vi "NI-Digital Burst I2C.vi"() -> ()   [LabVIEW 2024]
doc: "Overview\nDemonstrates how to use the NI-Digital Pattern Driver API to create and configure an instrument session and to burst a pattern on the digital pattern instrument using a start trigger."
uses:
  <instrlib>/niDigital/niDigital.llb/niDigital Write Static Pin State.ctl
  <instrlib>/niDigital/niDigital.llb/niDigital Selected Function.ctl
  <instrlib>/niDigital/niDigital.llb/niDigital Load Specifications Levels and Timing (Single).vi
  <instrlib>/niDigital/niDigital.llb/niDigital Write Source Waveform (Site Unique U32).vi
  <instrlib>/niDigital/niDigital.llb/niDigital Burst Pattern (Burst Only).vi
  <instrlib>/Semi Device Control/Utils/DIO Pin State.ctl
  <instrlib>/Semi Device Control/Semiconductor Device Control.lvclass
panel:
  in  "Tab Control":enum32{"SDC on", "Digital Low Level"}(tab)
  in  "Write SDC":bool
  in  "stop":bool
  in  "Register UID":string="CTRL_REG1"
  out "Register Value":u64
  in  "Write Value SDC":u64 format="%.0b"
  in  "Read SDC":bool
  in  "stop SDC":bool
  in  "Register Adress":u64 format="%.0x"
  out "Register Value Low Level":u32
  in  "Digital Pattern Resource":refnum<k15>="HSD_6571_C01_S02" caption="resource name"
  in  "Write Data":u64 format="%.0x"
  in  "Write Button LL":bool
  in  "Read Button LL":bool
  out "error out":errorcluster
  # "Overview\nDemonstrates how to use the NI-Digital Pattern Driver API to create and configure an instrument session and to burst a pattern on the digital pattern instrument using a start trigger.\n\nInstructions\n1. Use the resource name control to select the digital pattern instrument. Ensure that the instrument name in the PinMap.pinmap file matches the resource name of the digital pattern instrument. The default value for the resource name is \"PXI1Slot2,PXI1Slot3\".\n2. Use the start trigger mode tab control to select the start trigger mode to use. The active tab determines the configured start trigger at run time. Some tabs include additional configuration options.\n3. Run the VI.\n4. To run on hardware deselect Simulate?  and modify the resource name as appropriate."
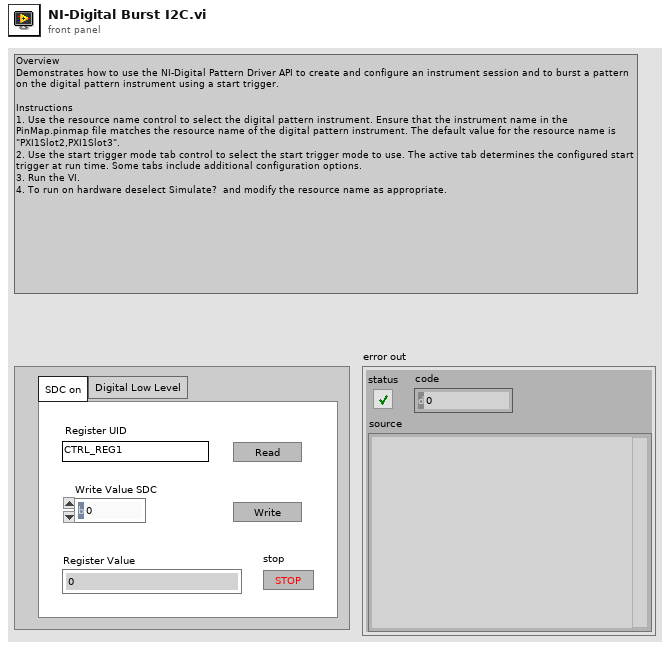
[diagram p1: front panel]
types:
  T1 = typedef "Semiconductor Device Control.lvclass/DIO Pin State.ctl" = enum16{"Low", "High", "Term"}
  T2 = typedef "niDigital Write Static Pin State.ctl" = u8
  T3 = typedef "niDigital Selected Function.ctl" = i32
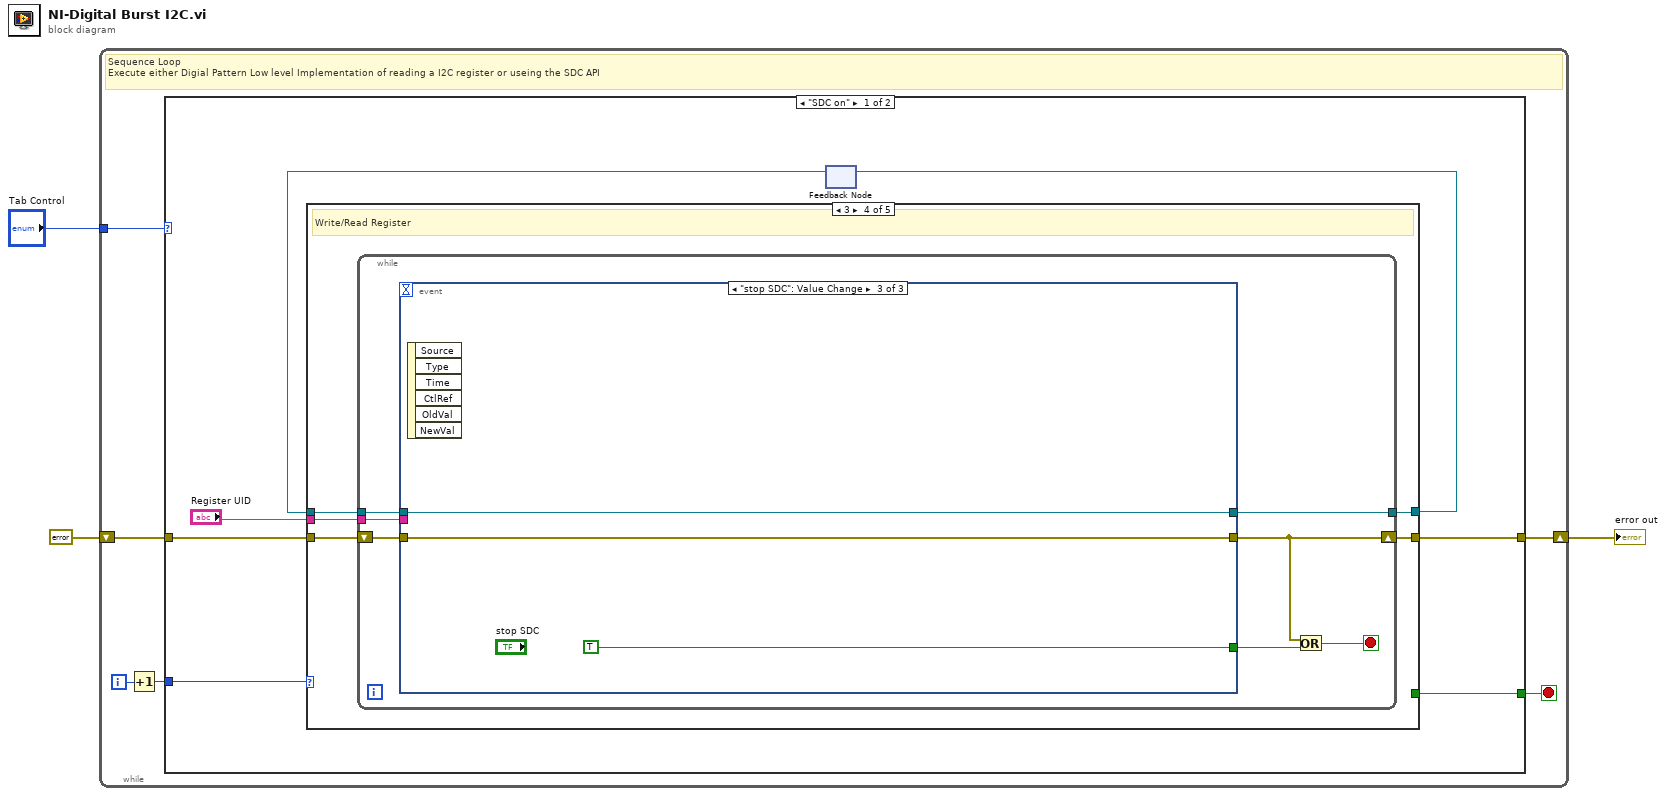
[diagram p0: block diagram]
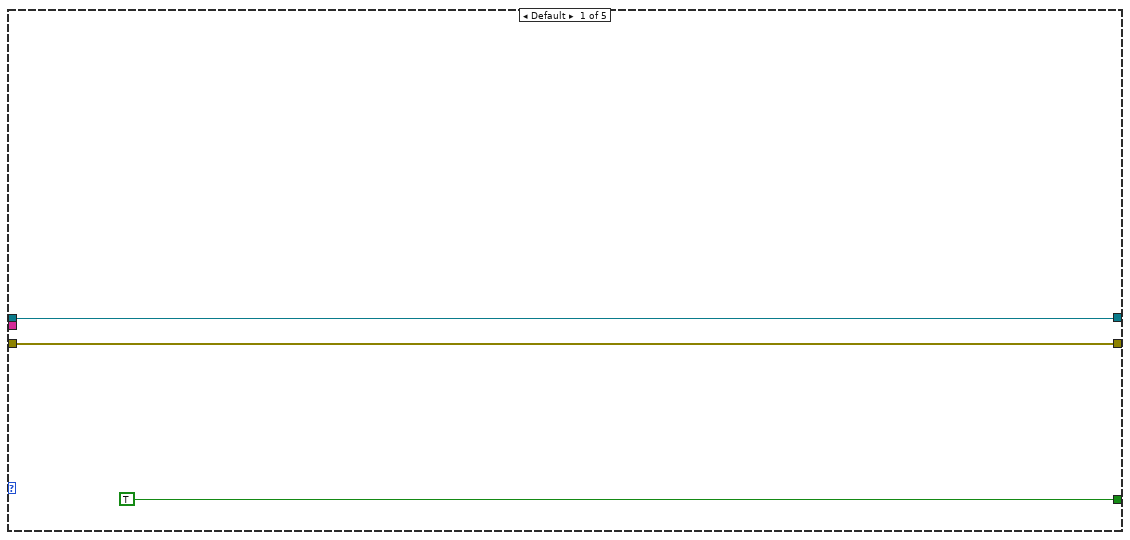
[diagram p2: hidden frame]
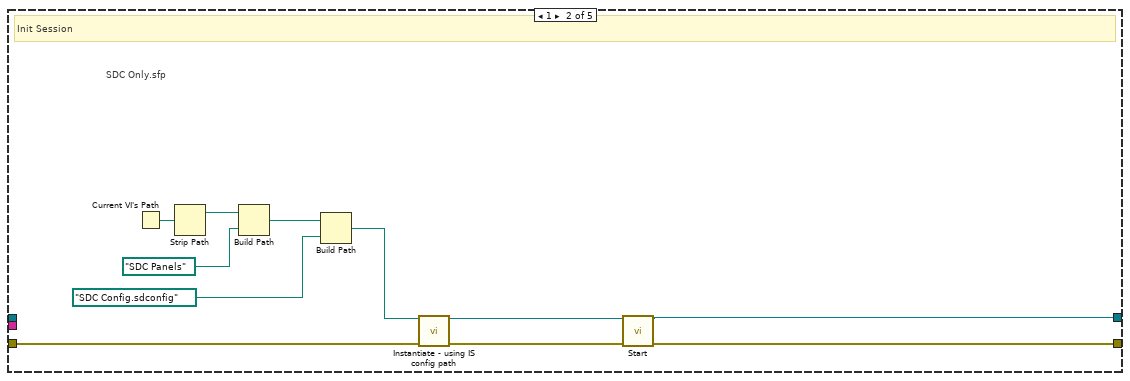
[diagram p3: hidden frame]
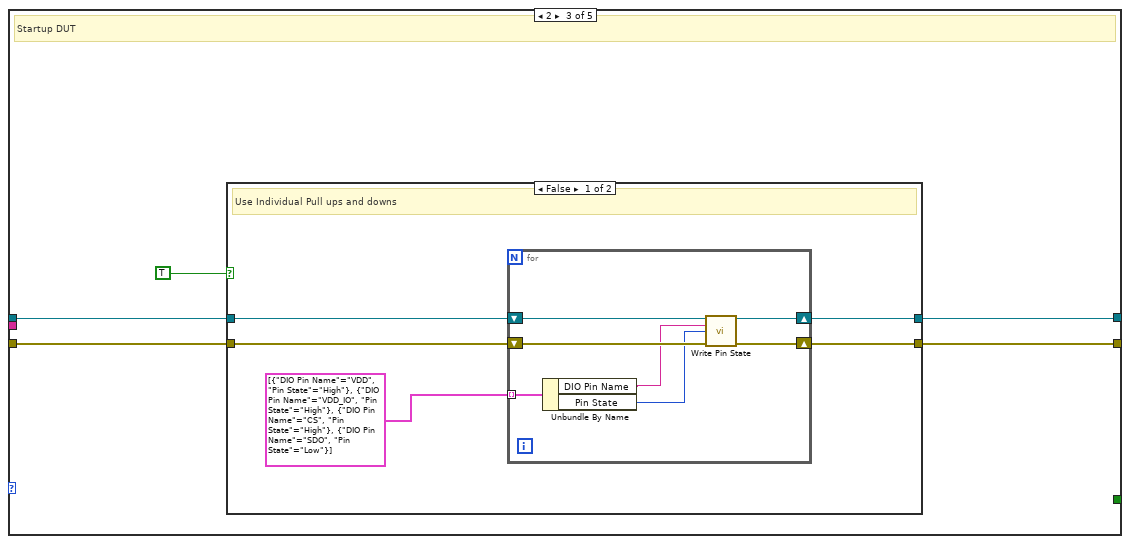
[diagram p4: hidden frame]
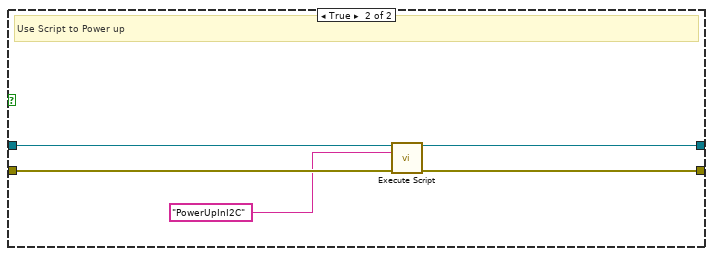
[diagram p5: hidden frame]
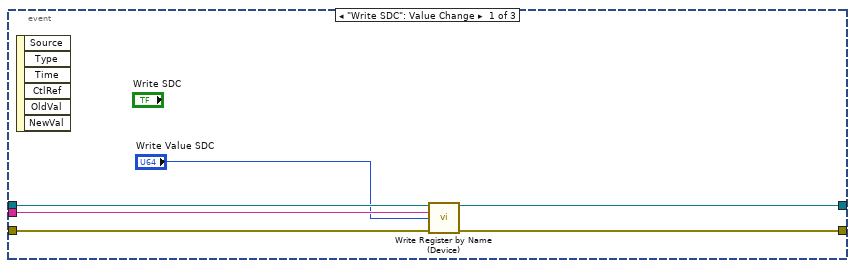
[diagram p6: hidden frame]
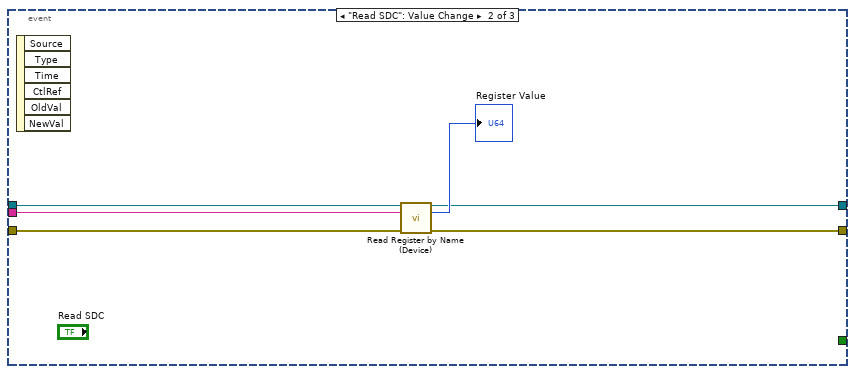
[diagram p7: hidden frame]
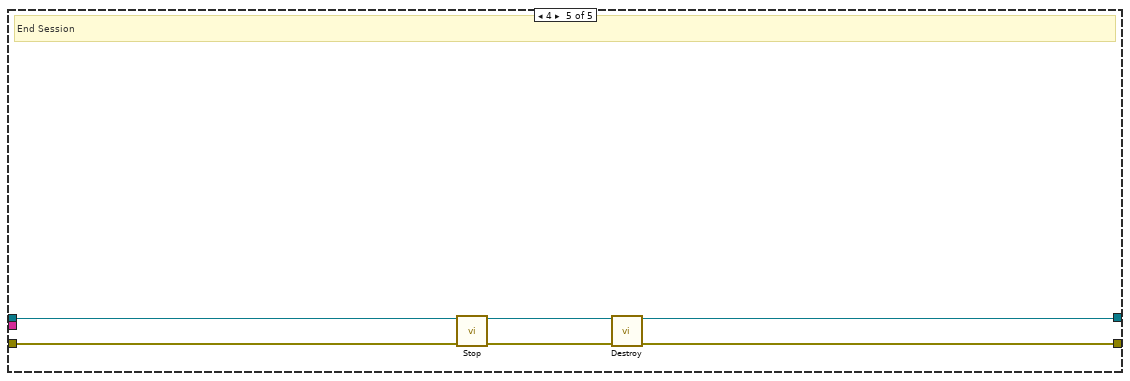
[diagram p8: hidden frame]
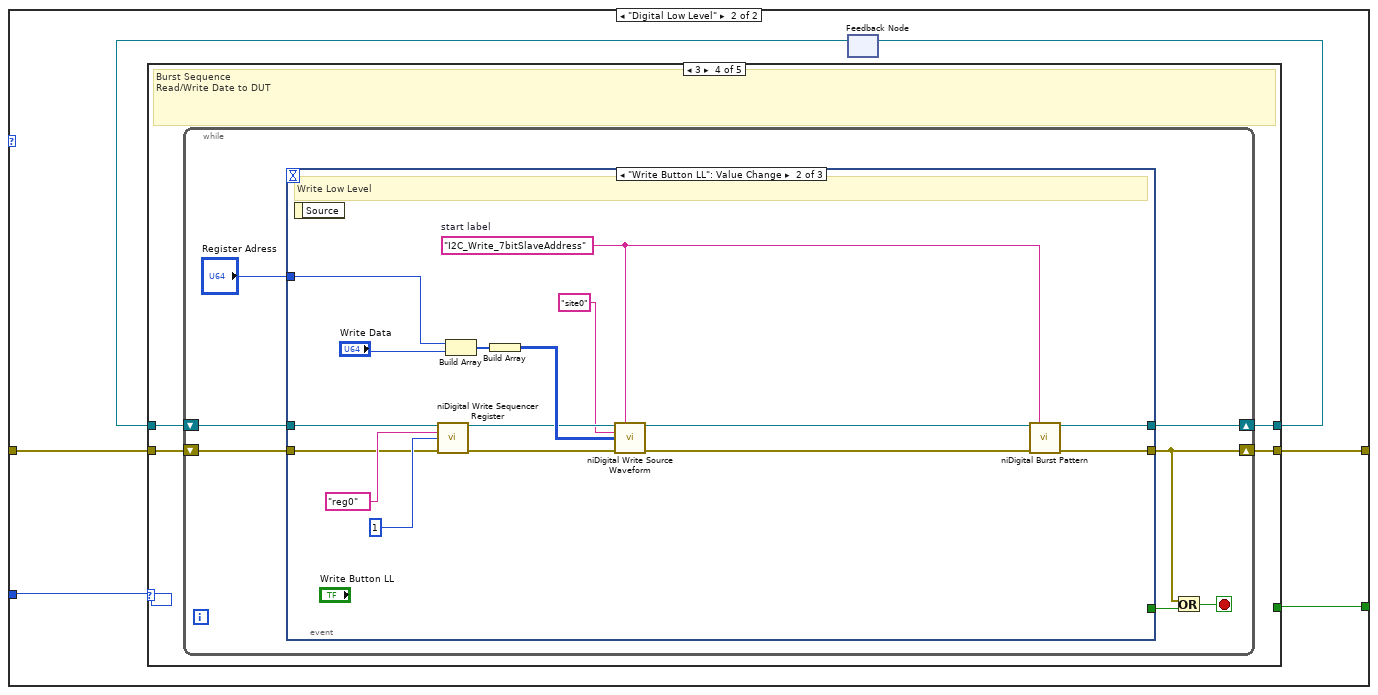
[diagram p9: hidden frame]
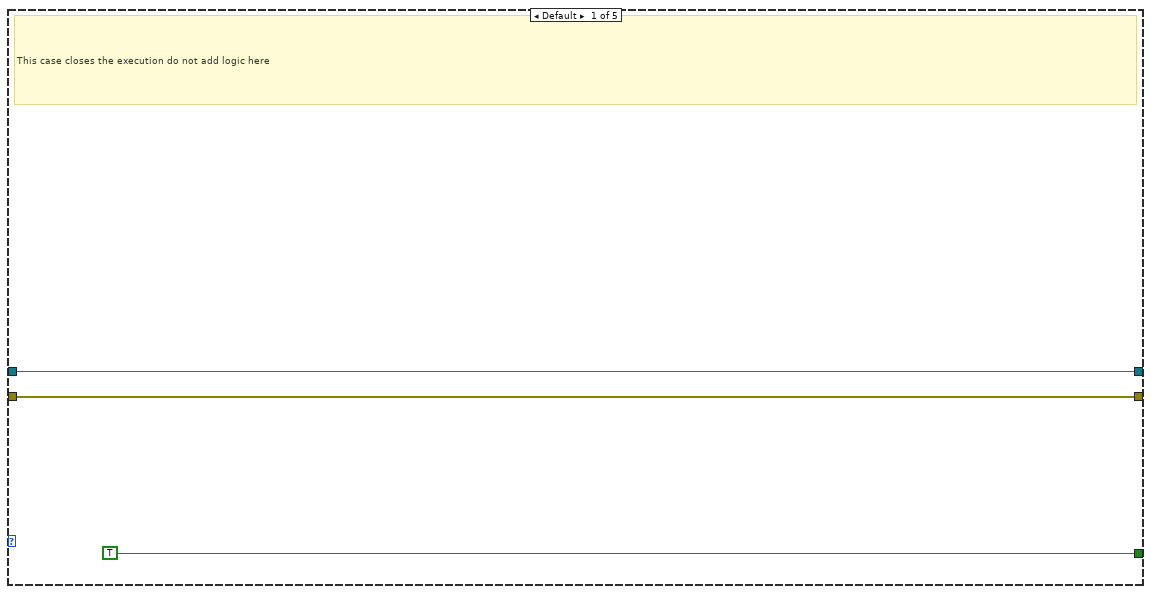
[diagram p10: hidden frame]
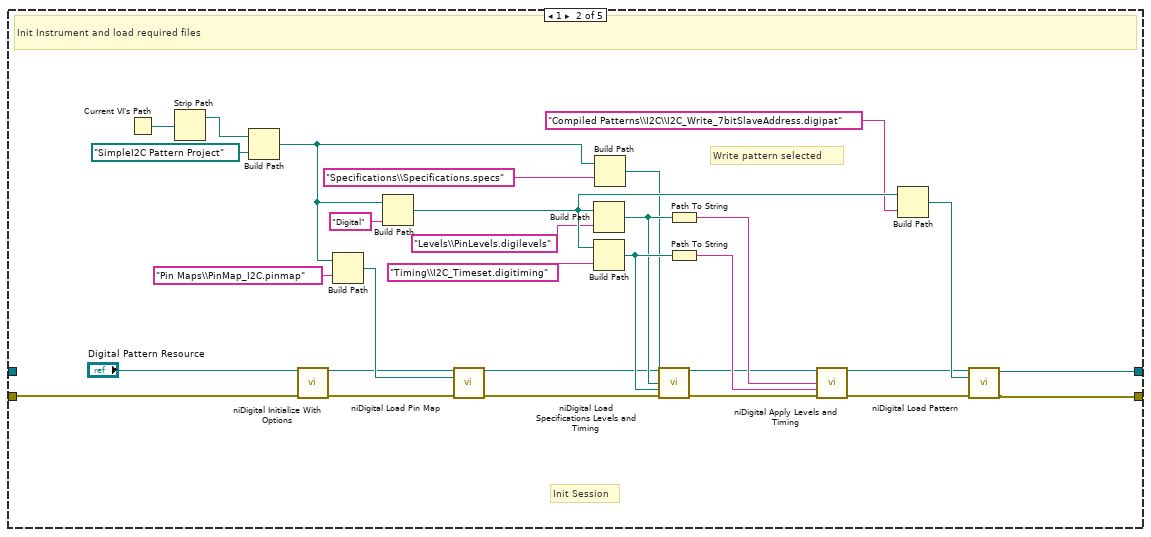
[diagram p11: hidden frame]
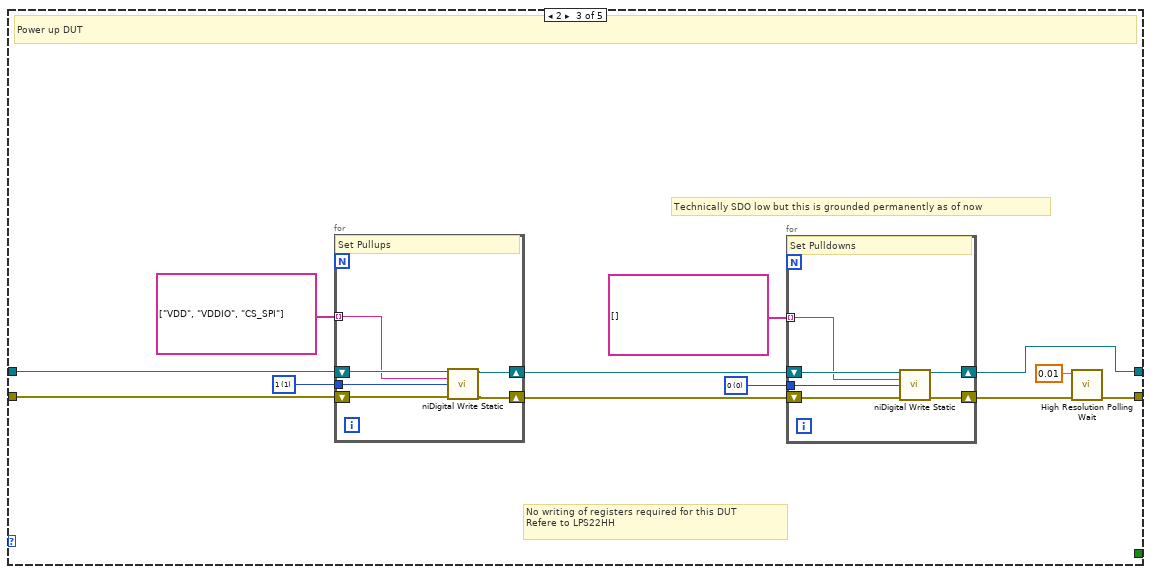
[diagram p12: hidden frame]
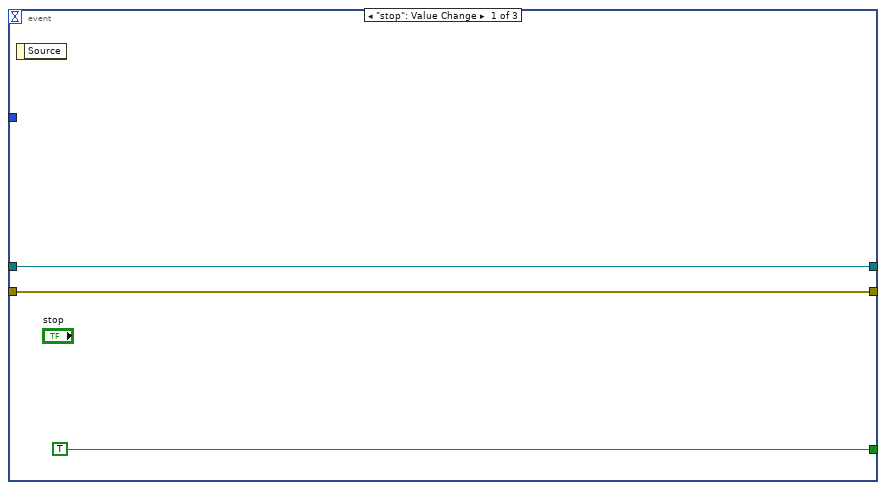
[diagram p13: hidden frame]
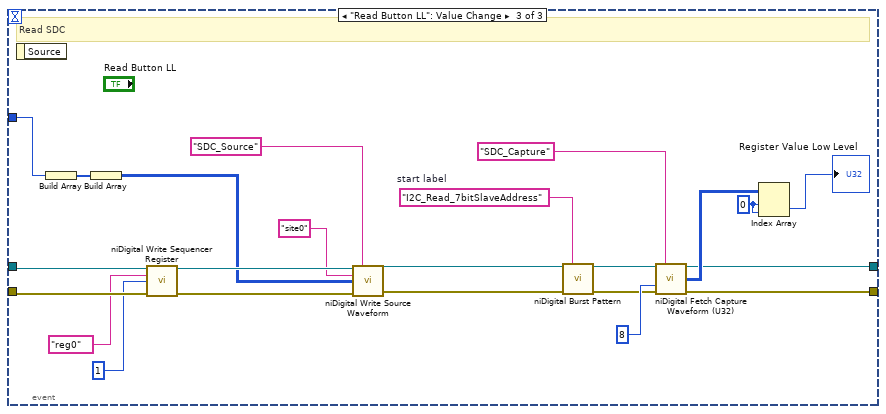
[diagram p14: hidden frame]
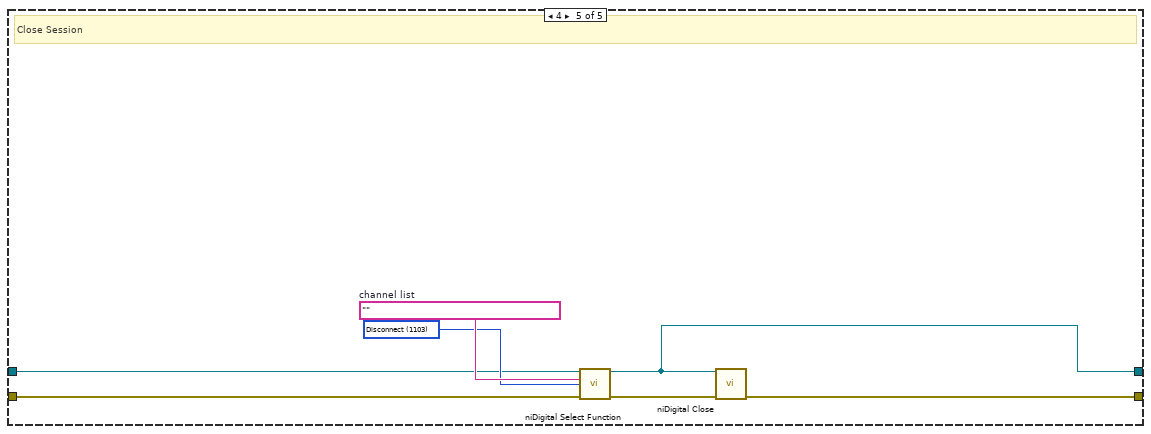
[diagram p15: hidden frame]
diagram:
  n1 = while {
    shift-right: [w8] -> w3
    shift-left: errorcluster {"status"=FALSE, "code"=0, "source"=""} ("error out") -> [w9]
    tunnel: "Tab Control" -> [w4]
    i -> [w6]
    stop <- w7 stop-if-true
    # "Sequence Loop\nExecute either Digial Pattern Low level Implementation of reading a I2C register or useing the SDC API"
    n2 = Increment(x=w6) -> (x+1=w5:i32)
    n3 = case shown="\"SDC on\"" w4 {
      tunnel: w9 -> [w14 w91]
      tunnel: [w13 w90] -> w8
      tunnel: [w15 w89] -> w7
      tunnel: w5 -> [w16 w88]
      frame "SDC on" {
        n4 = feedback #1() -> (w11:refnum<class "Semiconductor Device Control.lvclass">)  [unwired: 1 in]
        n5 = case shown="3" w16 {
          tunnel: [TRUE _ _ _ _] -> w15
          tunnel: w14 -> [w18 w30 w35 w57 w83]
          tunnel: [w18 w27 w34 w56 w81] -> w13
          tunnel: w11 -> [w17 _ w33 w54 w82]
          tunnel: [w17 w26 w32 w55 w80] -> w12
          tunnel: "Register UID" -> [_ _ _ w53 _]
          frame Default {
          }
          frame 1 {
            # "SDC Only.sfp"
            # "Init Session"
            n6 = Current VI's Path() -> (path=w25:path)
            n7 = Strip Path(path=w25) -> (stripped path=w24:path)  [unwired: 1 out]
            n8 = Build Path(base path=w24, name or relative path=path "SDC Panels") -> (appended path=w22:path)
            n9 = Build Path(base path=w22, name or relative path=path "SDC Config.sdconfig") -> (appended path=w21:path)
            n10 = call <instrlib>:"Instantiate - using IS config path.vi"("IS Semi Device Control config path"=w21, "error in (no error)"=w30) -> ("Device Control session out"=w29:refnum<class "Semiconductor Device Control.lvclass">, "error out"=w28:errorcluster)  [unwired: 12 in]
            n11 = call <instrlib>:"Start.vi"("Device Control session in"=w29, "error in (no error)"=w28) -> ("Device Control session out"=w26:refnum<class "Semiconductor Device Control.lvclass">, "error out"=w27:errorcluster)  [unwired: 12 in]
          }
          frame 2 {
            # "Startup DUT"
            n12 = case shown="False" TRUE {
              tunnel: w35 -> [w40 w52]
              tunnel: [w39 w51] -> w34
              tunnel: w33 -> [w38 w50]
              tunnel: [w37 w49] -> w32
              frame False {
                # "Use Individual Pull ups and downs"
                n13 = for {
                  shift-right: [w46] -> w39
                  shift-left: w40 -> [w47]
                  shift-right: [w44] -> w37
                  shift-left: w38 -> [w45]
                  tunnel: cluster{"DIO Pin Name":string, "Pin State":T1}[] [{"DIO Pin Name"="VDD", "Pin State"=enum."High"}, {"DIO Pin Name"="VDD_IO", "Pin State"=enum."High"}, {"DIO Pin Name"="CS", "Pin State"=enum."High"}, {"DIO Pin Name"="SDO", "Pin State"=enum."Low"}] -> [w43] mode=indexing
                  n14 = Unbundle By Name(w43) -> ("DIO Pin Name"=w42:string, "Pin State"=w41:T1)
                  n15 = call <instrlib>:"Write Pin State.vi"("Device Control session in"=w45, "DIO Pin Name"=w42, "Pin State"=w41, "error in (no error)"=w47) -> ("Device Control session out"=w44:refnum<class "Semiconductor Device Control.lvclass">, "error out"=w46:errorcluster)  [unwired: 10 in]
                }
              }
              frame True {
                # "Use Script to Power up"
                n16 = call <instrlib>:"Execute Script.vi"("Device Control session in"=w50, "Script Name"="PowerUpInI2C", "error in"=w52) -> ("Device Control session out"=w49:refnum<class "Semiconductor Device Control.lvclass">, "error out"=w51:errorcluster)  [unwired: 10 in, 1 out]
              }
            }
          }
          frame 3 {
            # "Write/Read Register"
            n17 = while {
              tunnel: [w63] -> w55
              tunnel: w54 -> [w62]
              tunnel: w53 -> [w61]
              shift-right: [w60] -> w56
              shift-left: w57 -> [w64]
              stop <- w58 stop-if-true
              n18 = event shown="[2] \"stop SDC\": Value Change" {
                selector: _ -> [_ _ _]
                dyn-events: _ -> [_ _ _]
                timeout: _ -> [_ _ _]
                tunnel: w64 -> [w70 w71 w79]
                tunnel: [w69 w72 w79] -> w60
                tunnel: [w68 w75 w78] -> w63
                tunnel: w62 -> [w67 w74 w78]
                tunnel: w61 -> [w66 w73 _]
                tunnel: [_ _ TRUE ("stop SDC")] -> w59
                event "Write SDC": Value Change {
                  n19 = event-data() -> ()  [unwired: 1 in, 6 out]
                  n20 = call <instrlib>:"Write Register by Name (Device).vi"("Device Control session in"=w67, "Register UID"=w66, "Register Data"="Write Value SDC", "error in (no error)"=w70) -> ("Device Control session out"=w68:refnum<class "Semiconductor Device Control.lvclass">, "error out"=w69:errorcluster)  [unwired: 10 in]
                }
                event "Read SDC": Value Change {
                  n21 = event-data() -> ()  [unwired: 1 in, 6 out]
                  n22 = call <instrlib>:"Read Register by Name (Device).vi"("Device Control session in"=w74, "Register UID"=w73, "error in (no error)"=w71) -> ("Device Control session out"=w75:refnum<class "Semiconductor Device Control.lvclass">, "Register Data"=→"Register Value":u64, "error out"=w72:errorcluster)  [unwired: 10 in]
                }
                event "stop SDC": Value Change {
                  n23 = event-data() -> ()  [unwired: 1 in, 6 out]
                }
              }
              n24 = Or(x=w60, y=w59) -> (x .or. y?=w58:bool)
            }
          }
          frame 4 {
            # "End Session"
            n25 = call <instrlib>:"Stop.vi"("Device Control session in"=w82, "error in (no error)"=w83) -> ("Device Control session out"=w84:refnum<class "Semiconductor Device Control.lvclass">, "error out"=w85:errorcluster)  [unwired: 12 in]
            n26 = call <instrlib>:"Destroy.vi"("Device Control session in"=w84, "error in (no error)"=w85) -> ("Device Control session out"=w80:refnum<class "Semiconductor Device Control.lvclass">, "error out"=w81:errorcluster)  [unwired: 12 in]
          }
        }
        n27 = feedback-in #1(w12) -> ()
      }
      frame "Digital Low Level" {
        n28 = feedback #2() -> (w87:refnum<k15>)  [unwired: 1 in]
        n29 = case shown="3" w88 {
          tunnel: [w92 w99 w125 w152 w202] -> w86
          tunnel: w87 -> [w92 _ w135 w151 w204]
          tunnel: w91 -> [w93 w102 w136 w150 w205]
          tunnel: [w93 w101 w133 w149 w203] -> w90
          tunnel: [TRUE _ _ _ _] -> w89
          frame Default {
            # "This case closes the execution do not add logic here"
          }
          frame 1 {
            # "Write pattern selected"
            # "Init Session"
            # "Init Instrument and load required files"
            n30 = Current VI's Path() -> (path=w98:path)
            n31 = Strip Path(path=w98) -> (stripped path=w96:path)  [unwired: 1 out]
            n32 = Build Path(base path=w96, name or relative path=path "SimpleI2C Pattern Project") -> (appended path=w95:path)
            n33 = call <instrlib>:"niDigital Initialize With Options.vi"("resource name"="Digital Pattern Resource", "error in"=w102) -> ("instrument handle"=w114:refnum<k15>, "error out"=w115:errorcluster)  [unwired: 12 in]
            n34 = Build Path(base path=w95, name or relative path="Pin Maps\\PinMap_I2C.pinmap") -> (appended path=w119:path)
            n35 = Build Path(base path=w95, name or relative path="Digital") -> (appended path=w124:path)
            n36 = call <instrlib>:"niDigital Load Pin Map.vi"("instrument handle"=w114, "pin map file"=w119, "error in"=w115) -> ("instrument handle out"=w117:refnum<k15>, "error out"=w118:errorcluster)  [unwired: 11 in]
            n37 = Build Path(base path=w124, name or relative path="Levels\\PinLevels.digilevels") -> (appended path=w122:path)
            n38 = Build Path(base path=w124, name or relative path="Timing\\I2C_Timeset.digitiming") -> (appended path=w123:path)
            n39 = Build Path(base path=w95, name or relative path="Specifications\\Specifications.specs") -> (appended path=w121:path)
            n40 = call-poly <instrlib>:"niDigital Load Specifications Levels and Timing.vi"("instrument handle"=w117, "specifications file path"=w121, "levels file path"=w122, "timing file path"=w123, "error in"=w118) -> ("instrument handle out"=w109:refnum<k15>, "error out"=w110:errorcluster)  [unwired: 9 in]
            n41 = Path To String(path=w122) -> (string=w116:string)
            n42 = Path To String(path=w123) -> (string=w113:string)
            n43 = call <instrlib>:"niDigital Apply Levels and Timing.vi"("instrument handle"=w109, "levels sheet"=w116, "timing sheet"=w113, "error in"=w110) -> ("instrument handle out"=w112:refnum<k15>, "error out"=w111:errorcluster)  [unwired: 10 in]
            n44 = Build Path(base path=w124, name or relative path="Compiled Patterns\\I2C\\I2C_Write_7bitSlaveAddress.digipat") -> (appended path=w120:path)
            n45 = call <instrlib>:"niDigital Load Pattern.vi"("instrument handle"=w112, "pattern file"=w120, "error in"=w111) -> ("instrument handle out"=w99:refnum<k15>, "error out"=w101:errorcluster)  [unwired: 11 in]
          }
          frame 2 {
            w129 = T2 0 items=["0"=0, "1"=1, "X"=5] ("state")
            w134 = T2 1 items=["0"=0, "1"=1, "X"=5] ("state")
            # "Technically SDO low but this is grounded permanently as of now"
            # "No writing of registers required for this DUT\nRefere to LPS22HH"
            # "Power up DUT"
            n46 = for {
              tunnel: w134 -> [w146]
              tunnel: string[] ["VDD", "VDDIO", "CS_SPI"] ("channel list") -> [w145] mode=indexing
              shift-right: [w144] -> w128
              shift-left: w135 -> [w147]
              shift-right: [w143] -> w127
              shift-left: w136 -> [w148]
              # "Set Pullups"
              n47 = call <instrlib>:"niDigital Write Static.vi"("instrument handle"=w147, "channel list"=w145, "state"=w146, "error in"=w148) -> ("instrument handle out"=w144:refnum<k15>, "error out"=w143:errorcluster)  [unwired: 10 in]
            }
            n48 = for {
              tunnel: w129 -> [w140]
              tunnel: string[] [] ("channel list") -> [w139] mode=indexing
              shift-right: [w138] -> w126
              shift-left: w127 -> [w142]
              shift-right: [w137] -> w125
              shift-left: w128 -> [w141]
              # "Set Pulldowns"
              n49 = call <instrlib>:"niDigital Write Static.vi"("instrument handle"=w141, "channel list"=w139, "state"=w140, "error in"=w142) -> ("instrument handle out"=w137:refnum<k15>, "error out"=w138:errorcluster)  [unwired: 10 in]
            }
            n50 = call <vilib>:"High Resolution Polling Wait.vi"("error in (no error)"=w126, "seconds to wait"=0.01) -> ("error out"=w133:errorcluster)  [unwired: 9 in]
          }
          frame 3 {
            # "Burst Sequence\nRead/Write Date to DUT"
            n51 = while {
              shift-right: [w155] -> w149
              shift-left: w150 -> [w157]
              shift-right: [w159] -> w152
              shift-left: w151 -> [w158]
              stop <- w153 stop-if-true
              n52 = event shown="[1] \"Write Button LL\": Value Change" {
                selector: _ -> [_ _ _]
                dyn-events: _ -> [_ _ _]
                timeout: _ -> [_ _ _]
                tunnel: [w161 w173 w197] -> w159
                tunnel: w158 -> [w161 w175 w194]
                tunnel: w157 -> [w162 w176 w195]
                tunnel: [w162 w174 w198] -> w155
                tunnel: [TRUE _ _] -> w154
                tunnel: "Register Adress" -> [_ w172 w189]
                event "stop": Value Change {
                  n53 = event-data() -> ()  [unwired: 1 in, 1 out]
                }
                event "Write Button LL": Value Change {
                  w164 = "I2C_Write_7bitSlaveAddress"  # start label
                  # "Write Low Level"
                  n54 = event-data() -> ()  [unwired: 1 in, 1 out]
                  n55 = call <instrlib>:"niDigital Write Sequencer Register.vi"("instrument handle"=w175, "sequencer register"="reg0", "value"=1, "error in"=w176) -> ("instrument handle out"=w168:refnum<k15>, "error out"=w166:errorcluster)  [unwired: 10 in]
                  n56 = Build Array(w172, "Write Data") -> (w170:u64[])
                  n57 = Build Array(w170) -> (w169:u64[][])
                  n58 = call-poly <instrlib>:"niDigital Write Source Waveform.vi"("instrument handle"=w168, "waveform name"=w164, "site list"="site0", "waveform data"=w169, "error in"=w166) -> ("instrument handle out"=w167:refnum<k15>, "error out"=w165:errorcluster)  [unwired: 9 in]
                  n59 = call-poly <instrlib>:"niDigital Burst Pattern.vi"("instrument handle"=w167, "start label"=w164, "error in"=w165) -> ("instrument handle out"=w173:refnum<k15>, "error out"=w174:errorcluster)  [unwired: 11 in]
                }
                event "Read Button LL": Value Change {
                  w200 = 0 ("index (row)")
                  w186 = "I2C_Read_7bitSlaveAddress"  # start label
                  # "Read SDC"
                  n60 = event-data() -> ()  [unwired: 1 in, 1 out]
                  n61 = Build Array(w189) -> (w188:u64[])
                  n62 = Build Array(w188) -> (w187:u64[][])
                  n63 = call <instrlib>:"niDigital Write Sequencer Register.vi"("instrument handle"=w194, "sequencer register"="reg0", "value"=1, "error in"=w195) -> ("instrument handle out"=w191:refnum<k15>, "error out"=w190:errorcluster)  [unwired: 10 in]
                  n64 = call-poly <instrlib>:"niDigital Write Source Waveform.vi"("instrument handle"=w191, "waveform name"="SDC_Source", "site list"="site0", "waveform data"=w187, "error in"=w190) -> ("instrument handle out"=w181:refnum<k15>, "error out"=w182:errorcluster)  [unwired: 9 in]
                  n65 = call-poly <instrlib>:"niDigital Burst Pattern.vi"("instrument handle"=w181, "start label"=w186, "error in"=w182) -> ("instrument handle out"=w185:refnum<k15>, "error out"=w184:errorcluster)  [unwired: 11 in]
                  n66 = call <instrlib>:"niDigital Fetch Capture Waveform (U32).vi"("instrument handle"=w185, "waveform name"="SDC_Capture", "samples to read"=8, "error in"=w184) -> ("instrument handle out"=w197:refnum<k15>, "data"=w201:u32[][], "error out"=w198:errorcluster)  [unwired: 9 in]
                  n67 = Index Array(array=w201, index (row)=w200, index (col)=w200) -> (element=→"Register Value Low Level":u32)
                }
              }
              n68 = Or(x=w155, y=w154) -> (x .or. y?=w153:bool)
            }
          }
          frame 4 {
            w207 = ""  # channel list
            w206 = T3 1103 items=["Digital"=1100, "PPMU"=1101, "Off"=1102, "Disconnect"=1103] ("function")
            # "Close Session"
            n69 = call <instrlib>:"niDigital Select Function.vi"("instrument handle"=w204, "channel list"=w207, "function"=w206, "error in"=w205) -> ("instrument handle out"=w202:refnum<k15>, "error out"=w208:errorcluster)  [unwired: 10 in]
            n70 = call <instrlib>:"niDigital Close.vi"("instrument handle"=w202, "error in"=w208) -> ("error out"=w203:errorcluster)  [unwired: 13 in]
          }
        }
        n71 = feedback-in #2(w86) -> ()
      }
    }
  }
  "error out" <- w3
